vi "Variable@KeyValue__Parameter.vi"(1 "ParamterIn":string) -> (0 "ParamterOut":string)   [LabVIEW 2020]
panel:
  in  "Section":string(combo)
  in  "Value":string(combo)
  in  "ParameterName":string(combo)
  in  "Confirm":bool
  # "Variable@KeyValue $Variable(@Section),$Value\n$Value can be string, number, 0xffff, or [ a; b; c; d;........] for List\nVariable can use this expression in IOLogic:\nvariable==NULL/EXIST\nUse $Variable or $(Variable) to parser in the command parameter"
  # "@"
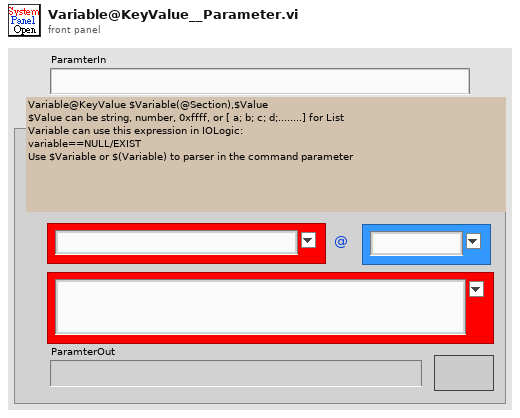
[diagram p1: front panel]
types:
  T1 = enum16{"Get", "Init", "Set", "Delete", "GetElement", "Inc", "Dec"}
  T2 = enum16{"Get", "Init", "Set", "Delete", "GetElement", "Inc", "Dec", "ReName"}
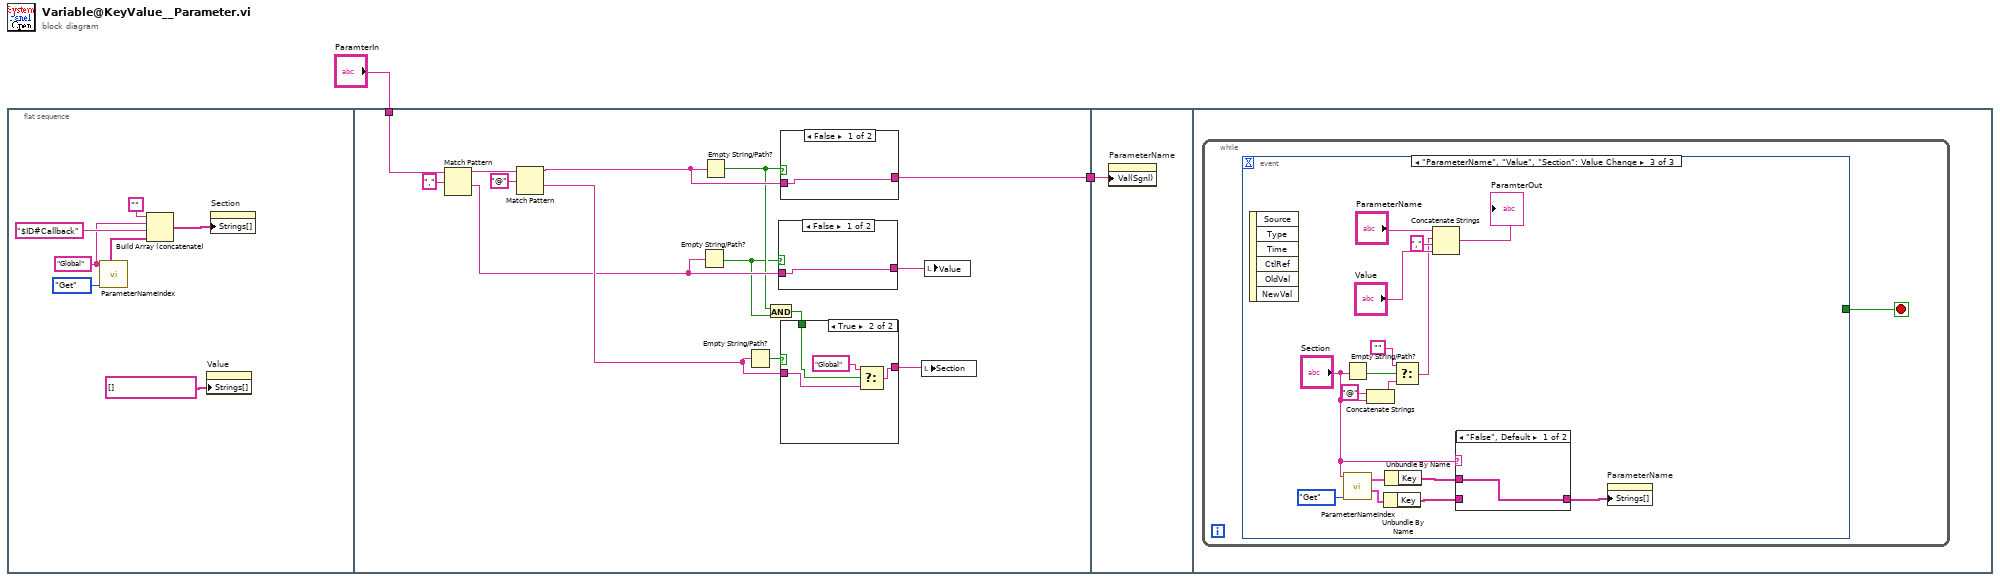
[diagram p0: block diagram]
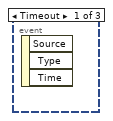
[diagram p5: hidden frame]
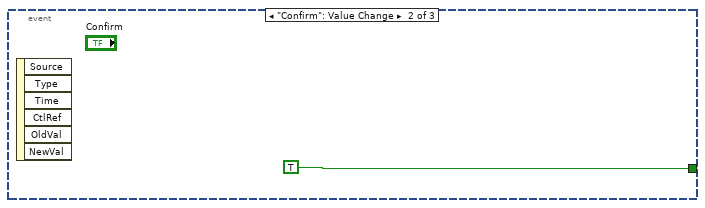
[diagram p6: hidden frame]
diagram:
  n1 = flat-sequence {
    tunnel: "ParamterIn" -> [w19]
    tunnel: [w23] -> w1
    tunnel: w1 -> [w33]
    frame #0 {
      w3 = "Global" ("VariableSection")
      n2 = call "ParameterNameIndex.vi"("OP"=T1."Get", "VariableSection"=w3) -> ("SectionList"=w7:string[])  [unwired: 3 in, 6 out]
      n3 = Build Array (concatenate)("", w3, "$ID#Callback" ("VariableSection"), w7) -> (w6:string[])
      n4 = property on="Value" class="CmbBox"("Strings[]"=string[] [] ("Strings []")) -> ()  [unwired: 2 in, 2 out]
      n5 = property on="Section" class="CmbBox"("Strings[]"=w6) -> ()  [unwired: 2 in, 2 out]
    }
    frame #1 {
      n6 = Match Pattern(string=w19, regular expression=",") -> (before substring=w17:string, after substring=w13:string)  [unwired: 1 in, 2 out]
      n7 = Match Pattern(string=w17, regular expression="@") -> (before substring=w15:string, after substring=w14:string)  [unwired: 1 in, 2 out]
      n8 = Empty String/Path?(string/path=w13) -> (empty?=w11:bool)
      n9 = Empty String/Path?(string/path=w15) -> (empty?=w12:bool)
      n10 = Empty String/Path?(string/path=w14) -> (empty?=w21:bool)
      n11 = And(x=w12, y=w11) -> (x .and. y?=w10:bool)
      n12 = case shown="False" w11 {
        tunnel: w13 -> [w29 w30]
        tunnel: [w29 w30] -> w22
        frame False {
        }
        frame True {
        }
      }
      n13 = case shown="False" w12 {
        tunnel: w15 -> [w31 w32]
        tunnel: [w31 w32] -> w23
        frame False {
        }
        frame True {
        }
      }
      n14 = case shown="True" w21 {
        tunnel: w14 -> [w24 w27]
        tunnel: [w24 w26] -> w20
        tunnel: w10 -> [_ w25]
        frame False {
        }
        frame True {
          n15 = Select(t="Global", s=w25, f=w27) -> (s? t:f=w26:string)
        }
      }
      n16 = local write "Section"(w20) -> ()
      n17 = local write "Value"(w22) -> ()
    }
    frame #2 {
      n18 = property on="ParameterName" class="CmbBox"("Val(Sgnl)"=w33) -> ()  [unwired: 2 in, 2 out]
    }
    frame #3 {
      n19 = while {
        stop <- w34 stop-if-true
        n20 = event shown="[2] \"ParameterName\", \"Value\", \"Section\": Value Change" {
          selector: _ -> [_ _ _]
          dyn-events: _ -> [_ _ _]
          timeout: _ -> [_ _ _]
          tunnel: [_ TRUE _] -> w34
          event Timeout {
            n21 = event-data() -> ()  [unwired: 1 in, 3 out]
          }
          event "Confirm": Value Change {
            n22 = event-data() -> ()  [unwired: 1 in, 6 out]
          }
          event "ParameterName", "Value", "Section": Value Change {
            n23 = event-data() -> ()  [unwired: 1 in, 6 out]
            n24 = Empty String/Path?(string/path="Section") -> (empty?=w45:bool)
            n25 = call "ParameterNameIndex.vi"("OP"=T2."Get", "VariableSection"="Section") -> ("GlobalKeyValue"=w44:cluster{"Key":string[], "Value":string[]}, "SectionKeyValue"=w46:cluster{"Key":string[], "Value":string[]})  [unwired: 3 in, 5 out]
            n26 = Concatenate Strings("@" ("string"), "Section") -> (w39:string)
            n27 = Unbundle By Name(w44) -> ("Key"=w43:string[])
            n28 = Unbundle By Name(w46) -> ("Key"=w41:string[])
            n29 = Select(t="", s=w45, f=w39) -> (s? t:f=w36:string)
            n30 = Concatenate Strings("ParameterName", w36, "," ("string"), "Value") -> (→"ParamterOut":string)
            n31 = case shown="\"False\", Default" "Section" {
              tunnel: w43 -> [_ w53]
              tunnel: [w52 w53] -> w42
              tunnel: w41 -> [w52 _]
              frame "False", Default {
              }
              frame "", "Global" {
              }
            }
            n32 = property on="ParameterName" class="CmbBox"("Strings[]"=w42) -> ()  [unwired: 2 in, 2 out]
          }
        }
      }
    }
  }
